vi "FGV - Login Status.vi"(6 "Action":enum16{"Read", "Write"}(ring)=enum."Write", 8 "Error In":errorcluster, 10 "Username in":string, 11 "Login In":bool) -> (0 "Error Out":errorcluster, 2 "Username Out":string, 3 "Login?":bool)   [LabVIEW 2020]
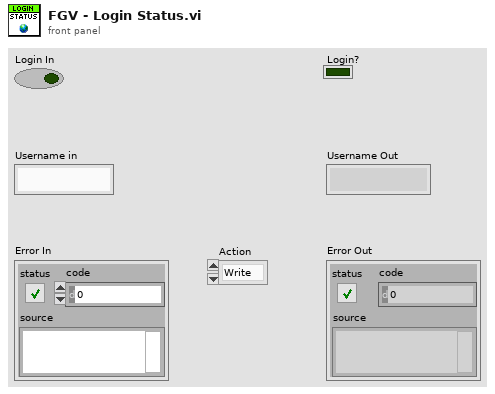
[diagram p1: front panel]
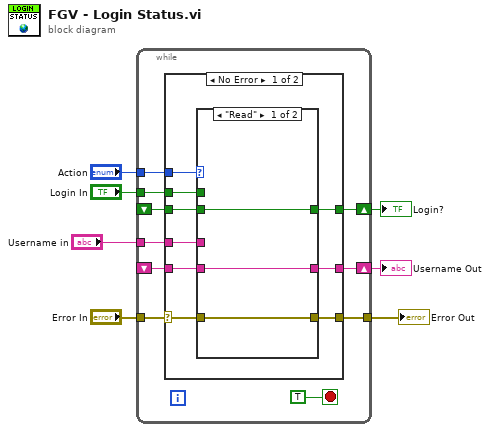
[diagram p0: block diagram]
diagram:
  n1 = while {
    tunnel: "Error In" -> [w17]
    tunnel: [w16] -> w6
    tunnel: "Action" -> [w14]
    tunnel: "Login In" -> [w13]
    shift-right: [w12] -> w3
    shift-left: _ -> [w11]
    tunnel: "Username in" -> [w9]
    shift-right: [w10] -> w1
    shift-left: _ -> [w8]
    stop <- TRUE stop-if-true
    n2 = case shown="No Error" w17 {
      selector: w17 -> [w26 w35]
      tunnel: [w25 w35] -> w16
      tunnel: w14 -> [w24 _]
      tunnel: w13 -> [w23 _]
      tunnel: [w22 w34] -> w12
      tunnel: w11 -> [w21 w34]
      tunnel: [w20 w33] -> w10
      tunnel: w9 -> [w19 _]
      tunnel: w8 -> [w18 w33]
      frame No Error {
        n3 = case shown="\"Read\"" w24 {
          tunnel: w26 -> [w29 w32]
          tunnel: w23 -> [_ w31]
          tunnel: [w29 w32] -> w25
          tunnel: [w28 w31] -> w22
          tunnel: w21 -> [w28 _]
          tunnel: [w27 w30] -> w20
          tunnel: w19 -> [_ w30]
          tunnel: w18 -> [w27 _]
          frame "Read" {
          }
          frame "Write" {
          }
        }
      }
      frame Error {
      }
    }
  }
  "Error Out" <- w6
  "Login?" <- w3
  "Username Out" <- w1
